vi "Connect.vi"(8 "error in":errorcluster, 11 "7976A in":refnum<class "7976A.lvclass">) -> (0 "error out":errorcluster, 3 "7976A out":refnum<class "7976A.lvclass">)   [LabVIEW 2019, in "7976A.lvlib" / "7976A.lvclass"]
uses:
  Library/7976A.lvclass
  C:/Users/Public/Documents/Development/builds/Instruments/Instruments.lvlibp/Library/Instruments.lvclass
  Library/7976A.lvclass/7976A.ctl
  builds/Instruments/Instruments.lvlibp/Accessors/Read Resource.vi
  builds/Engine/Engine.lvlibp/Project/Engine.lvclass
  <instrlib>/Agilent N7976A/Agilent N7976A.lvlib
  C:/Users/Public/Documents/Development/builds/Engine/Engine.lvlibp/Project/Engine.lvclass
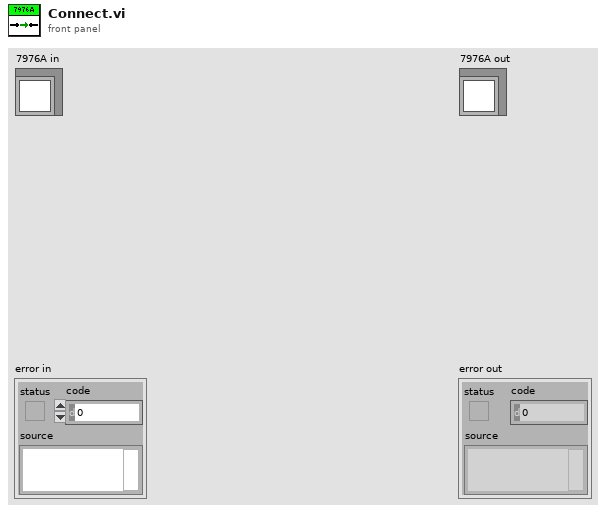
[diagram p1: front panel]
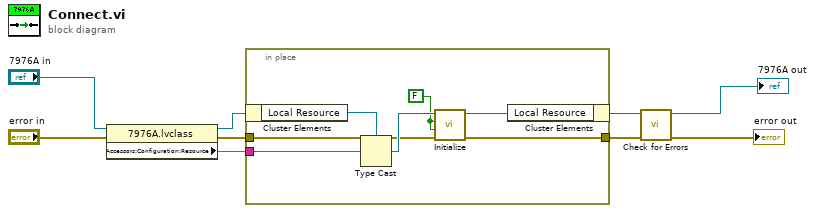
[diagram p0: block diagram]
diagram:
  n1 = property class="7976A.lvclass"(reference="7976A in", error in="error in") -> (reference out=w7:refnum<class "7976A.lvclass">, error out=w6:errorcluster, "Accessors:Configuration:Resource"=w8:string)
  n2 = in-place {
    in-place-border: w8 -> [w15]
    in-place-border: w6 -> [w12]
    in-place-border: [w11] -> w3
    w10 = FALSE ("ID Query (True)")
    n3 = in-place-cluster #1(w7) -> ("Local Resource"=w16:refnum<visa-resource-name>)
    n4 = Type Cast(type=w16, x=w15) -> (*(type *) &x=w13:refnum<visa-resource-name>)
    n5 = call <instrlib>:"Initialize.vi"("error in (no error)"=w12, "Reset (True)"=w10, "ID Query (True)"=w10, "VISA resource name"=w13) -> ("error out"=w11:errorcluster, "VISA resource name out"=w14:refnum<visa-resource-name>)  [unwired: 6 in]
    n6 = in-place-cluster #1("Local Resource"=w14) -> (w4:refnum<class "7976A.lvclass">)
  }
  n7 = call "Check for Errors.vi"("error in"=w3, "Engine in"=w4) -> ("error out"=→"error out":errorcluster, "Engine out"=→"7976A out":refnum<class "7976A.lvclass">)  [unwired: 8 in]
